vi "TempestUDP.vi"() -> ()   [LabVIEW 2021]
doc: "Use this VI with the UDP Sender VI. Run this VI first.\n\nThe UDP protocol differs from TCP in that there is no error-checking with the packets of information that are sent, and thus no guarantee whatsoever that an intended recipient will actually receive a given piece of data.\n\nUDP does offer the ability to \"broadcast\" data across a network--simply specify an IP Address of all ones (255.255.255.255) to attempt to broadcast information network-wide. Keep in mind that routers and other network hardware will generally refuse to forward the broadcast beyond certain points, so the extent of the broadcast will in practice be limited."
panel:
  out "concatenated string":string
  out "length":i32
  out "Array - String":T1(array[cluster]) {"Time Stamp" format="%<%Y-%m-%d\n%H:%M:%S>T"}
  in  "timeout(ms)":i32=200
  out "error out":errorcluster
  out "loop":i32
  in  "max bytes/read":i32=548
  in  "Port":u16=50222
  in  "stop":bool
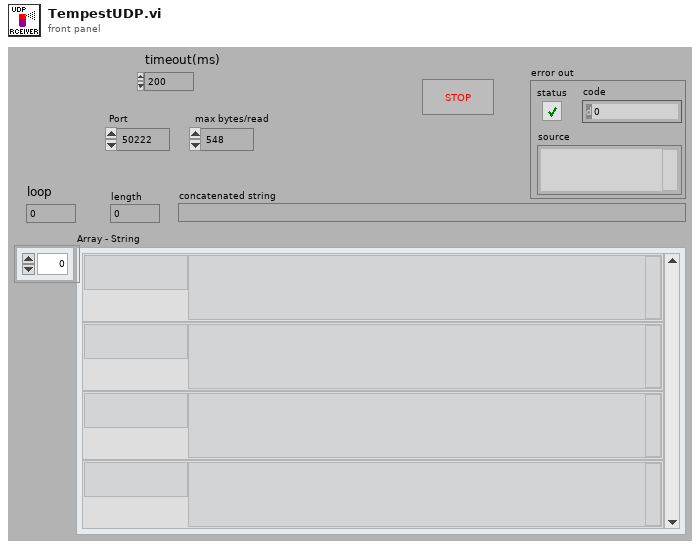
[diagram p1: front panel]
types:
  T1 = cluster{"Time Stamp":timestamp, "String":string}[]
  T2 = cluster{"seconds since 1Jan1904":timestamp, "data out":string}[]
  T3 = cluster{"seconds since 1Jan1904":timestamp, string}
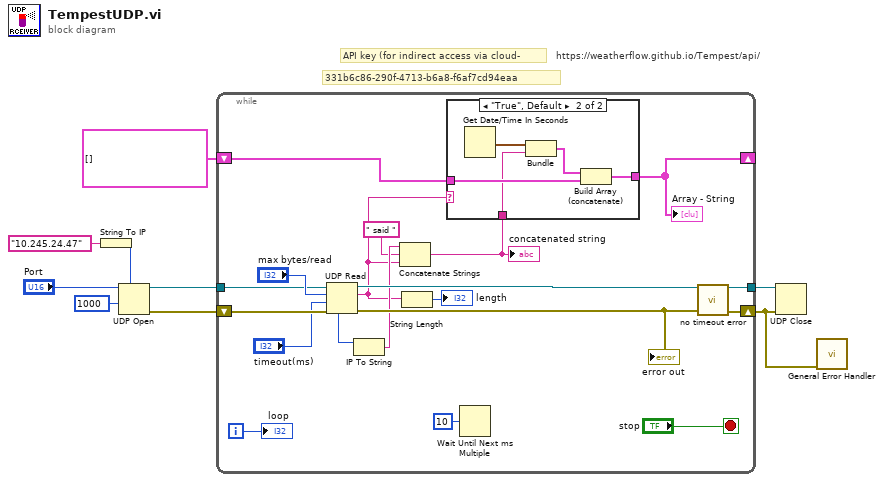
[diagram p0: block diagram]
diagram:
  # "https://weatherflow.github.io/Tempest/api/"
  # "API key (for indirect access via cloud-"
  # "331b6c86-290f-4713-b6a8-f6af7cd94eaa"
  n1 = String To IP(1:"10.245.24.47" ("name")) -> (0:w2:u32)
  n2 = UDP Open(7:w2, 9:1000 ("timeout ms (25000)"), 11:"Port") -> (port=w8:refnum<k16>, 0:w9:errorcluster)  [unwired: 2 in, 1 out]
  n3 = while {
    tunnel: [w27] -> w7
    tunnel: w8 -> [w21]
    shift-left: w9 -> [w20]
    shift-right: [w25] -> w5
    shift-right: [w17] -> _
    shift-left: T2 [] -> [w18]
    i -> [w23]
    stop <- "stop" stop-if-true
    n4 = UDP Read(connection ID=w21, max size (548)="max bytes/read", timeout ms (25000)="timeout(ms)", 8:w20) -> (data out=w12:string, error out=w26:errorcluster, 3:w27:refnum<k16>, 6:w16:u32)  [unwired: 1 out]
    "error out" <- w26
    n5 = IP To String(2:w16) -> (0:w15:string)  [unwired: 1 in]
    n6 = Concatenate Strings(w15, " said ", w12) -> (w13:string)
    "concatenated string" <- w13
    n7 = String Length(string=w12) -> (length=→"length":i32)
    n8 = case shown="\"True\", Default" w12 {
      tunnel: w18 -> [w28 w33]
      tunnel: [w28 w30] -> w17
      tunnel: w13 -> [_ w29]
      frame "\u0000" {
      }
      frame "True", Default {
        n9 = Get Date/Time In Seconds() -> (seconds since 1Jan1904=w32:timestamp)
        n10 = Bundle("seconds since 1Jan1904"=w32, w29) -> (w31:T3)  [unwired: 1 in]
        n11 = Build Array (concatenate)(w31, w33) -> (w30:T2)
      }
    }
    "Array - String" <- w17
    n12 = Wait Until Next ms Multiple(millisecond multiple=u32 10) -> ()  [unwired: 1 out]
    n13 = call "no timeout error.vi"("error in (no error)"=w26) -> ("error out"=w25:errorcluster)
    "loop" <- w23
  }
  n14 = UDP Close(connection ID=w7, 8:w5) -> ()  [unwired: 2 out]
  n15 = call <vilib>:"General Error Handler.vi"("error in (no error)"=w5) -> ()  [unwired: 10 in, 5 out]
